vi "Decode Status Byte.vi"(2 "Window Mode Notifier":refnum<notifier>, 3 "Status":T1) -> (0 "Status":T2(ring), 1 "Mode":enum8{"Tele-Op", "Auto", "Test", ""}(ring)=enum."Test")   [LabVIEW 2012]
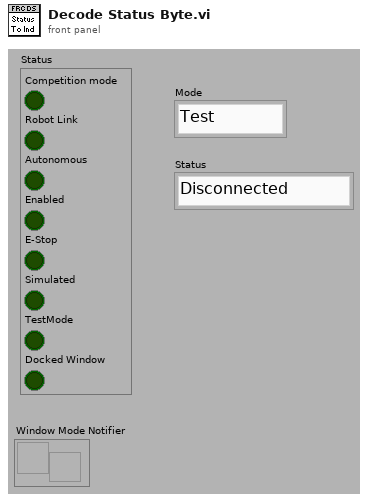
[diagram p1: front panel]
types:
  T1 = cluster{"Competition mode":bool, "Robot Link":bool, "Autonomous":bool, "Enabled":bool, "E-Stop":bool, "Simulated":bool, "TestMode":bool, "Docked Window":bool}
  T2 = enum8{"Disconnected", "E-Stop", "Disabled", "Enabled"}
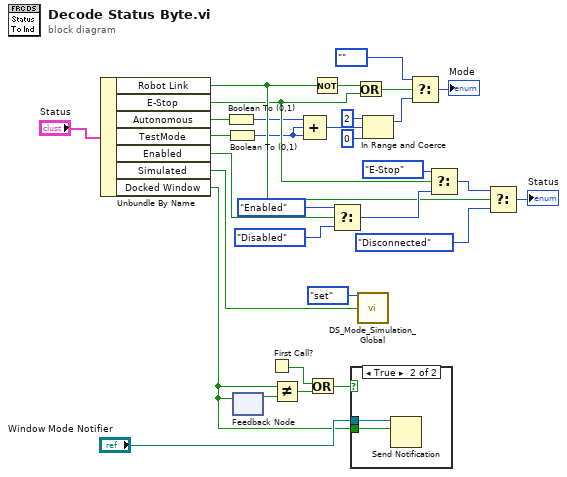
[diagram p0: block diagram]
diagram:
  n1 = Unbundle By Name("Status") -> ("Robot Link"=w24:bool, "E-Stop"=w17:bool, "Autonomous"=w20:bool, "TestMode"=w16:bool, "Enabled"=w15:bool, "Simulated"=w1:bool, "Docked Window"=w4:bool)
  n2 = Boolean To (0,1)(Boolean=w20) -> (0, 1=w14:i16)
  n3 = Boolean To (0,1)(Boolean=w16) -> (0, 1=w13:i16)
  n4 = feedback-in #1(w4) -> ()
  n5 = feedback #1() -> (w8:bool)  [unwired: 1 in]
  n6 = First Call?() -> (First Call?: T/F=w6:bool)
  n7 = Not Equal?(x=w4, y=w8) -> (x != y?=w7:bool)
  n8 = Compound Arithmetic op=ADD(w14, w13, w13) -> (w12:i16)
  n9 = Or(x=w6, y=w7) -> (x .or. y?=w3:bool)
  n10 = Not(x=w24) -> (.not. x?=w19:bool)
  n11 = Select(t=T2."Enabled" ("Status"), s=w15, f=T2."Disabled" ("Status")) -> (s? t:f=w29:T2)
  n12 = case shown="True" w3 {
    tunnel: "Window Mode Notifier" -> [_ w33]
    tunnel: w4 -> [_ w32]
    frame False {
    }
    frame True {
      n13 = Send Notification(notification=w32, notifier=w33) -> ()  [unwired: 1 in, 2 out]
    }
  }
  n14 = Or(x=w19, y=w17) -> (x .or. y?=w21:bool)
  n15 = call <vilib>:"DS_Mode_Simulation_Global.vi"("menu"=enum16{"set", "get"}."set", "simulated? in"=w1) -> ()  [unwired: 12 in, 2 out]
  n16 = In Range and Coerce(upper limit=i16 2, x=w12, lower limit=i16 0) -> (coerced(x)=w9:i16)  [unwired: 1 out]
  n17 = Select(t=enum8{"Tele-Op", "Auto", "Test", ""}."" ("Mode"), s=w21, f=w9) -> (s? t:f=→"Mode":i16)
  n18 = Select(t=T2."E-Stop" ("Status"), s=w17, f=w29) -> (s? t:f=w27:T2)
  n19 = Select(t=w27, s=w24, f=T2."Disconnected" ("Status")) -> (s? t:f=→"Status":T2)
